vi "test Deploy Scripted Custom Device with Additional Properties.vi"(8 "error in (no error)":errorcluster, 11 "TestCase in":refnum<class "Embedded Data Logger Scripting System Tests.lvclass">) -> (0 "error out":errorcluster, 3 "TestCase out":refnum<class "Embedded Data Logger Scripting System Tests.lvclass">)   [LabVIEW 2027, in "Embedded Data Logger Scripting System Tests.lvclass"]
uses:
  Embedded Data Logger Scripting System Tests.lvclass
  Embedded Data Logger Scripting System Tests.lvclass/Embedded Data Logger Scripting System Tests.ctl
  <vilib>/addons/_JKI Toolkits/VI Tester/TestCase.llb/TestCase.lvclass
  30dc589a-39cd-48ac-8e8d-4a58a160e88c.vi
  <vilib>/NI/VeriStand Custom Device Testing Tools/VeriStandTestUtilities/VeriStandTestUtilities.lvlib
  Embedded Data Logger Scripting.lvlib
  C:/NetCoreDLL/NationalInstruments.VeriStand.SystemDefinitionAPI.dll
  NetCoreDLL/NationalInstruments.VeriStand.SystemDefinitionAPI.dll
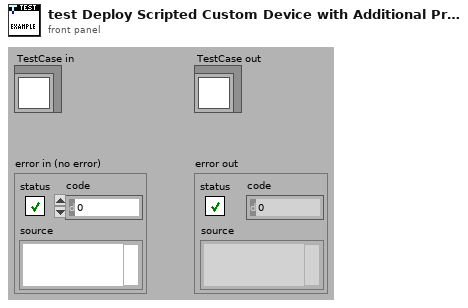
[diagram p1: front panel]
types:
  T1 = typedef "Custom Device API.lvlib/Custom Device Item Ref.ctl" = u64
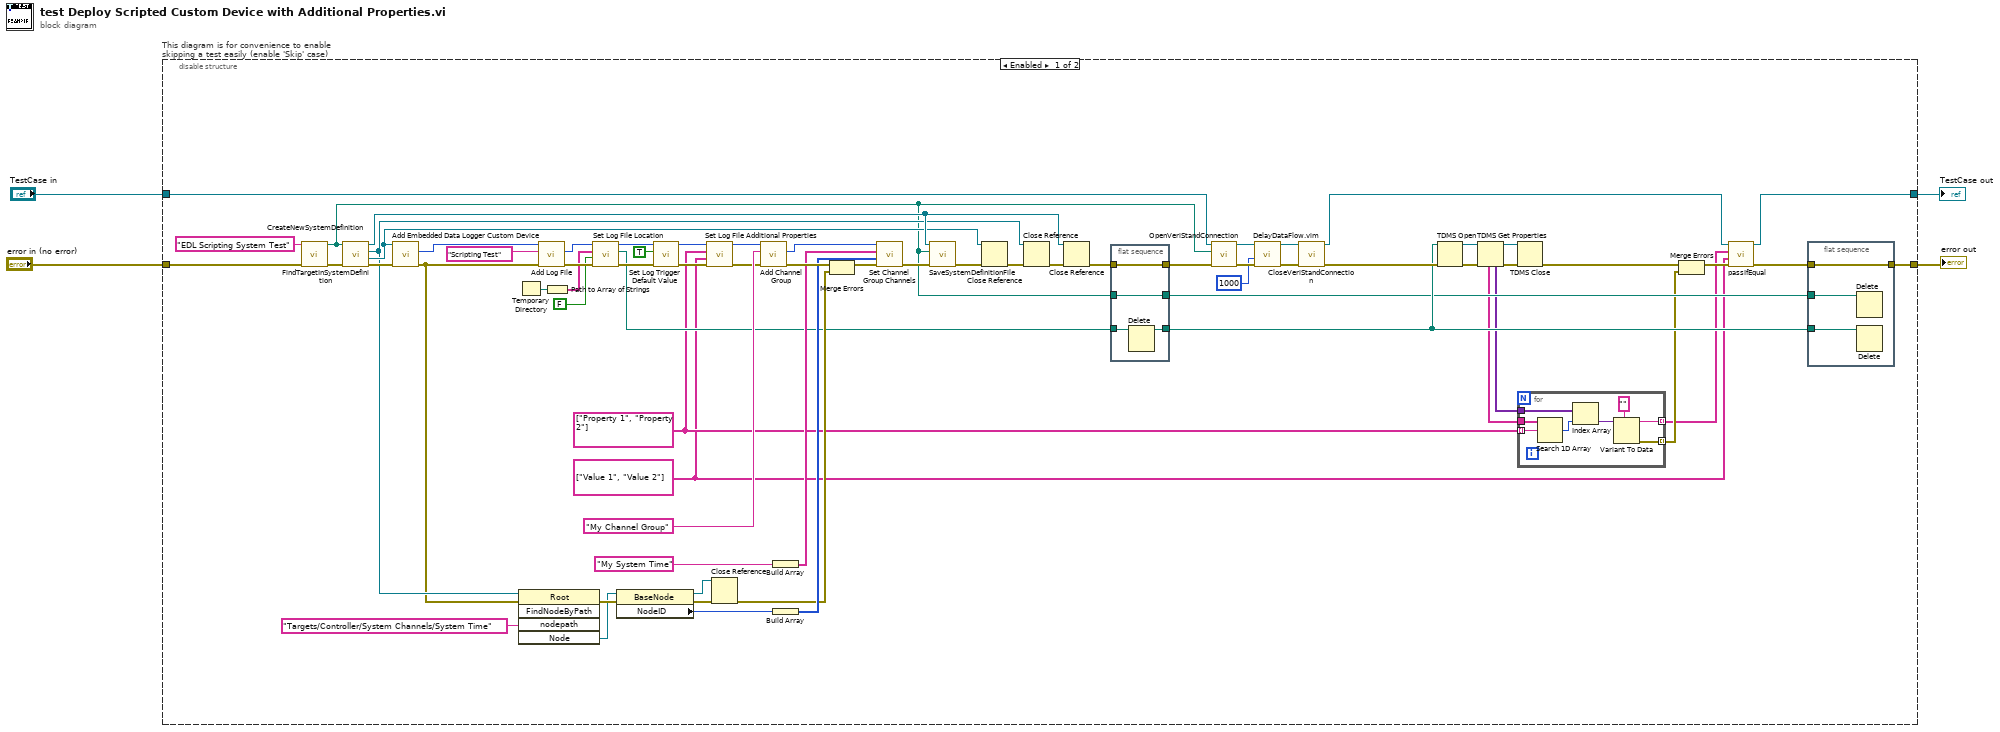
[diagram p0: block diagram]
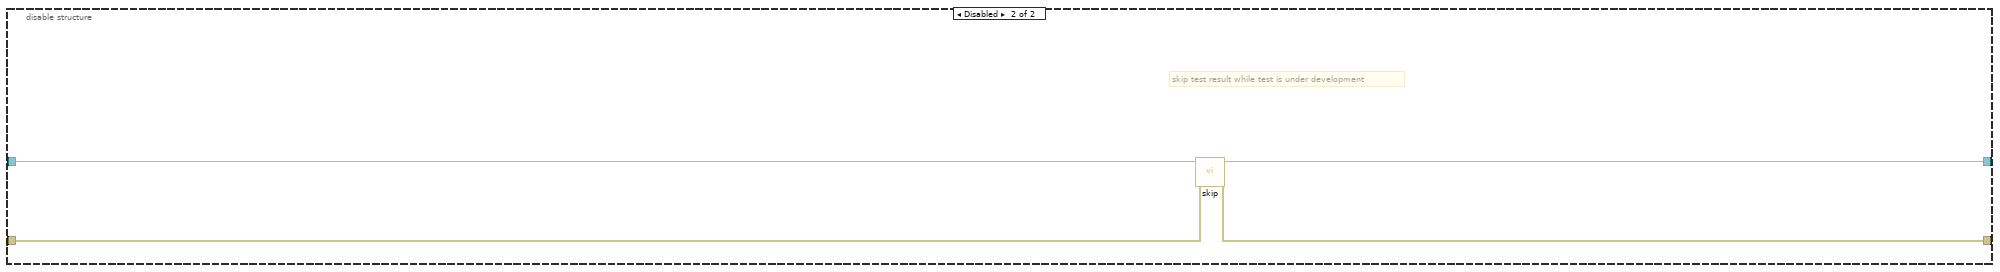
[diagram p2: hidden frame]
diagram:
  n1 = disable-structure "This diagram is for convenience to enable skipping a test easily (enable 'Skip' case)" shown="Enabled" {
    disable-tunnel: "TestCase in" -> [w72 w91]
    disable-tunnel: [w15 w89] -> w1
    disable-tunnel: [w58 w90] -> w3
    disable-tunnel: "error in (no error)" -> [w67 w88]
    frame Enabled {
      w6 = string[] ["Value 1", "Value 2"] ("property values")
      w13 = string[] ["Property 1", "Property 2"] ("property names")
      n2 = call <vilib>:"CreateNewSystemDefinition.vi"("error in"=w67, "System Definition Name"="EDL Scripting System Test") -> ("error out"=w66:errorcluster, "System Definition Path"=w21:path)  [unwired: 8 in]
      n3 = call <vilib>:"FindTargetInSystemDefinition.vi"("error in"=w66, "system definition path"=w21) -> ("error out"=w63:errorcluster, "NationalInstruments.VeriStand.SystemDefinitionAPI.Target"=w45:refnum<k39>, "NationalInstruments.VeriStand.SystemDefinitionAPI.Root"=w37:refnum<k39>, "NationalInstruments.VeriStand.SystemDefinitionAPI.SystemDefinition"=w46:refnum<k39>)  [unwired: 6 in]
      n4 = call "Add Embedded Data Logger Custom Device.vi"("error in"=w63, "NationalInstruments.VeriStand.SystemDefinitionAPI.Target"=w45) -> ("error out"=w31:errorcluster, "embedded data logger"=w52:T1)  [unwired: 7 in, 1 out]
      n5 = Temporary Directory() -> (w59:path)
      n6 = invoke class="Root" method="FindNodeByPath"(reference=w37, error in=w31, "nodepath"="Targets/Controller/System Channels/System Time" ("Item Path in")) -> (error out=w36:errorcluster, "Node"=w35:refnum<k39>)  [unwired: 2 in, 3 out]
      n7 = call "Add Log File.vi"("error in"=w31, "log file name"="Scripting Test", "embedded data logger in"=w52) -> ("error out"=w62:errorcluster, "log file"=w29:T1)  [unwired: 6 in, 1 out]
      n8 = Path to Array of Strings(0:w59) -> (2:w61:string[])  [unwired: 1 out]
      n9 = call "Set Log File Location.vi"("error in"=w62, "timestamp file name"=FALSE, "directory parts"=w61, "log file in"=w29) -> ("error out"=w57:errorcluster, "sample path"=w25:path, "log file out"=w56:T1)  [unwired: 5 in]
      n10 = property class="BaseNode"(reference=w35, error in=w36) -> (reference out=w34:refnum<k39>, error out=w33:errorcluster, "NodeID"=w32:u64)
      n11 = call "Set Log Trigger Default Value.vi"("error in"=w57, "log trigger default value"=TRUE, "log file in"=w56) -> ("error out"=w19:errorcluster, "log file out"=w17:T1)  [unwired: 7 in]
      n12 = call "Set Log File Additional Properties.vi"("error in"=w19, "property values"=w6, "property names"=w13, "log file in"=w17) -> ("error out"=w18:errorcluster, "log file out"=w16:T1)  [unwired: 6 in]
      n13 = Close Reference(reference=w34, error in (no error)=w33) -> (error out=w30:errorcluster)
      n14 = call "Add Channel Group.vi"("error in"=w18, "group name"="My Channel Group", "log file in"=w16) -> ("error out"=w54:errorcluster, "channel group"=w28:T1)  [unwired: 6 in, 1 out]
      n15 = Build Array("My System Time" ("Item Path in")) -> (w26:string[])
      n16 = Build Array(w32) -> (w50:u64[])
      n17 = Merge Errors(w54, w30) -> (w51:errorcluster)
      n18 = call "Set Channel Group Channels.vi"("error in"=w51, "channels"=w50, "names"=w26, "channel group in"=w28) -> ("error out"=w53:errorcluster)  [unwired: 4 in, 3 out]
      n19 = call <vilib>:"SaveSystemDefinitionFile.vi"("error in (no error)"=w53, "System Definition File in"=w21, "NationalInstruments.VeriStand.SystemDefinitionAPI.SystemDefinition"=w46) -> ("error out"=w64:errorcluster)  [unwired: 7 in, 1 out]
      n20 = Close Reference(reference=w45, error in (no error)=w64) -> (error out=w47:errorcluster)
      n21 = Close Reference(reference=w37, error in (no error)=w47) -> (error out=w48:errorcluster)
      n22 = Close Reference(reference=w46, error in (no error)=w48) -> (error out=w22:errorcluster)
      n23 = flat-sequence {
        tunnel: w25 -> [w84]
        tunnel: [w83] -> w24
        tunnel: [w82] -> w23
        tunnel: w22 -> [w82]
        tunnel: w21 -> [w81]
        tunnel: [w81] -> w20
        frame #0 {
          n24 = Delete(path (use dialog)=w84) -> (deleted path=w83:path)  [unwired: 4 in, 2 out]
        }
      }
      n25 = call-dynamic "OpenVeriStandConnection.vi"("error in (no error)"=w23, "System Definition File"=w21, "VeriStand Test Case in"=w72) -> ("error out"=w70:errorcluster, "VeriStand Test Case out"=w71:refnum<class "Embedded Data Logger Scripting System Tests.lvclass">)  [unwired: 6 in, 1 out]
      n26 = call "DelayDataFlow.vim"("value in"=w70, "milliseconds to wait"=u32 1000) -> ("value out"=w69:errorcluster)  [unwired: 2 in, 1 out]
      n27 = call-dynamic "CloseVeriStandConnection.vi"("error in (no error)"=w69, "VeriStand Test Case in"=w71) -> ("error out"=w49:errorcluster, "VeriStand Test Case out"=w10:refnum<class "Embedded Data Logger Scripting System Tests.lvclass">)  [unwired: 8 in]
      n28 = TDMS Open(8:w49, 11:w24) -> (0:w43:errorcluster, 3:w40:refnum<k34>)  [unwired: 5 in]
      n29 = TDMS Get Properties(8:w43, 11:w40) -> (0:w41:errorcluster, 3:w39:refnum<k34>, 4:w12:variant[], 6:w14:string[])  [unwired: 4 in, 2 out]
      n30 = TDMS Close(8:w41, 11:w39) -> (0:w9:errorcluster)  [unwired: 1 out]
      n31 = for {
        tunnel: w14 -> [w80]
        tunnel: w13 -> [w79] mode=indexing
        tunnel: w12 -> [w78]
        tunnel: [w74] -> w5 mode=indexing
        tunnel: [w73] -> w7 mode=indexing
        n32 = Search 1D Array(1D array=w80, element=w79) -> (index of element=w77:i32)  [unwired: 1 in]
        n33 = Index Array(array=w78, index=w77) -> (element=w76:variant)
        n34 = Variant To Data(type="", Variant=w76) -> (data=w74:string, error out=w73:errorcluster)  [unwired: 1 in]
      }
      n35 = Merge Errors(w9, w7) -> (w8:errorcluster)
      n36 = call-dynamic "passIfEqual.vi"("error in (no error)"=w8, "y"=w6, "x"=w5, "TestCase in"=w10) -> ("error out"=w11:errorcluster, "TestCase out"=w15:refnum<class "Embedded Data Logger Scripting System Tests.lvclass">)  [unwired: 6 in]
      n37 = flat-sequence {
        tunnel: w20 -> [w85]
        tunnel: w24 -> [w87]
        tunnel: [w86] -> w58
        tunnel: w11 -> [w86]
        frame #0 {
          n38 = Delete(path (use dialog)=w85) -> ()  [unwired: 4 in, 3 out]
          n39 = Delete(path (use dialog)=w87) -> ()  [unwired: 4 in, 3 out]
        }
      }
    }
    frame Disabled {
      # "skip test result while test is under development"
      n40 = call <vilib>:"skip.vi"("error in (no error)"=w88, "TestCase in"=w91) -> ("error out"=w90:errorcluster, "TestCase out"=w89:refnum<class "Embedded Data Logger Scripting System Tests.lvclass">)  [unwired: 8 in]
    }
  }
  "error out" <- w3
  "TestCase out" <- w1
